vi "Move.vi"(9 "Team In":refnum<class "Team.lvclass">, 11 "Square in":refnum<class "Square.lvclass">) -> (1 "Team":refnum<class "Team.lvclass">, 3 "Square out":refnum<class "Square.lvclass">)   [LabVIEW 2020, in "SquareBattle.lvlib" / "Square.lvclass"]
doc: "This VI is called to let a square know it has successfully moved to a new location. It is still possible for the square to be eliminated due to another square moving, replicating into the position, or the position was attacked while the square moved into it."
uses:
  Square.lvclass
  Team/Team.lvclass
  Square.lvclass/Square.ctl
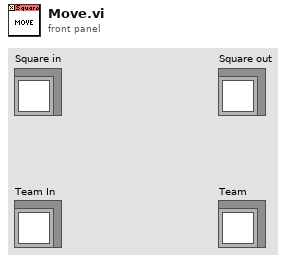
[diagram p1: front panel]
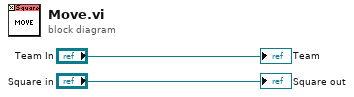
[diagram p0: block diagram]
diagram:
  "Square out" <- "Square in"
  "Team" <- "Team In"
